vi "Get Server Internal UEs.vi"(11 "OOP Server in":refnum<class "ctet_dio.lvclass">) -> (2 "Server Internal UEs":T1, 3 "OOP Server out":refnum<class "ctet_dio.lvclass">)   [LabVIEW 2019, in "ctet_dio.lvlib" / "ctet_dio.lvclass"]
uses:
  ctet_dio.lvclass
  typeDefs/Server Internal UEs.ctl
  typeDefs/Server Internal Message.ctl
  ctet_dio.lvclass/ctet_dio.ctl
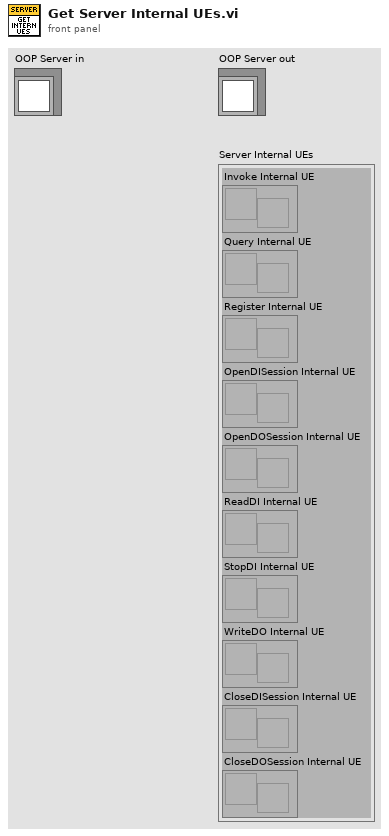
[diagram p1: front panel]
types:
  T1 = typedef "ctet_dio.lvlib/ctet_dio.lvclass/Server Internal UEs.ctl" = cluster{"Invoke Internal UE":refnum<user-event>, "Query Internal UE":refnum<user-event>, "Register Internal UE":refnum<user-event>, "OpenDISession Internal UE":refnum<user-event>, "OpenDOSession Internal UE":refnum<user-event>, "ReadDI Internal UE":refnum<user-event>, "StopDI Internal UE":refnum<user-event>, "WriteDO Internal UE":refnum<user-event>, "CloseDISession Internal UE":refnum<user-event>, "CloseDOSession Internal UE":refnum<user-event>}
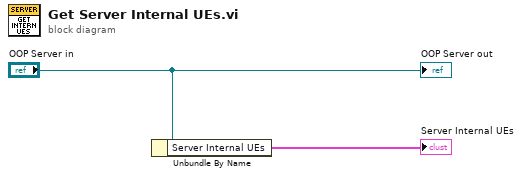
[diagram p0: block diagram]
diagram:
  n1 = Unbundle By Name("OOP Server in") -> ("Server Internal UEs"=→"Server Internal UEs":T1)
  "OOP Server out" <- "OOP Server in"
